vi "search instance list for class.vi"(10 "UID":string, 11 "instance data":T1[](array[typedef])) -> (3 "index":i32)   [LabVIEW 2023, in "CEF.lvlib"]
doc: "Searches a flattened instance set for a given class and returns the index of the first match.Copyright 2017 National Instruments Corporation\n\nLicensed under the Apache License, Version 2.0 (the \"License\"); you may not use this file except in compliance with the License. You may obtain a copy of the License at http://www.apache.org/licenses/LICENSE-2.0\nUnless required by applicable law or agreed to in writing, software distributed under the License is distributed on an \"AS IS\" BASIS, WITHOUT WARRANTIES OR CONDITIONS OF ANY KIND, either express or implied. See the License for the specific language governing permissions and limitations under the License."
uses:
  CEF.lvlib
  instance data.ctl
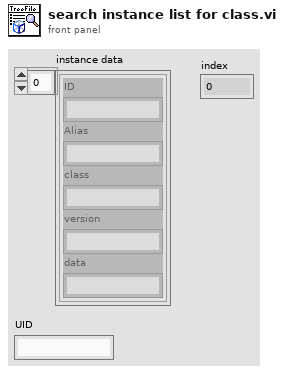
[diagram p1: front panel]
types:
  T1 = typedef "CEF.lvlib/instance data.ctl" = cluster{"ID":string, "Alias":string, "class":string, "version":string, "data":string}
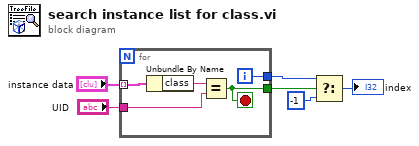
[diagram p0: block diagram]
diagram:
  n1 = for {
    tunnel: "instance data" -> [w8] mode=indexing
    tunnel: "UID" -> [w11]
    tunnel: [w10] -> w5
    tunnel: [w9] -> w6
    i -> [w10]
    stop <- w9 stop-if-true
    n2 = Unbundle By Name(w8) -> ("class"=w7:string)
    n3 = Equal?(x=w7, y=w11) -> (x = y?=w9:bool)
  }
  n4 = Select(t=w5, s=w6, f=-1) -> (s? t:f=→"index":i32)
